vi "Handle Error.vi"(8 "error in (no error)":errorcluster, 11 "Abstract Display Console in":refnum<class "Abstract Display Console.lvclass">) -> (0 "error out":errorcluster, 2 "stop actor?":bool=TRUE, 3 "Abstract Display Console out":refnum<class "Abstract Display Console.lvclass">)   [LabVIEW 2019, in "Abstract Display Console Actor.lvlib" / "Abstract Display Console.lvclass"]
doc: "(<B>Filename</B>: Actor Framework.lvlib:Actor.lvclass:Handle Error.vi)\n\nDefines how the actor handles an error that occurred while processing a message. By default, this method does nothing except stop the actor."
uses:
  Abstract Display Console.lvclass
  C:/Program Files (x86)/National Instruments/LabVIEW 2019/vi.lib/ActorFramework/Actor/Actor.lvclass
  <vilib>/ActorFramework/Actor/Actor.lvclass/Actor.ctl
  Elevator Controller Actor/Elevator Controller Messages/Centrize Error Handler Msg/Centrize Error Handler Msg.lvclass/Centrize Error Handler Msg.ctl
  <vilib>/ActorFramework/Message Enqueuer/Message Enqueuer.lvclass/Message Enqueuer.ctl
  <vilib>/ActorFramework/Message Enqueuer/Enqueue.vi
  Elevator Controller Actor/Elevator Controller Messages/Centrize Error Handler Msg/Centrize Error Handler Msg.lvclass
  C:/Program Files (x86)/National Instruments/LabVIEW 2019/vi.lib/ActorFramework/Message/Message.lvclass
  <vilib>/ActorFramework/Message Priority Queue/Priority Enqueue.vi
  <vilib>/ActorFramework/Actor/Actor.lvclass
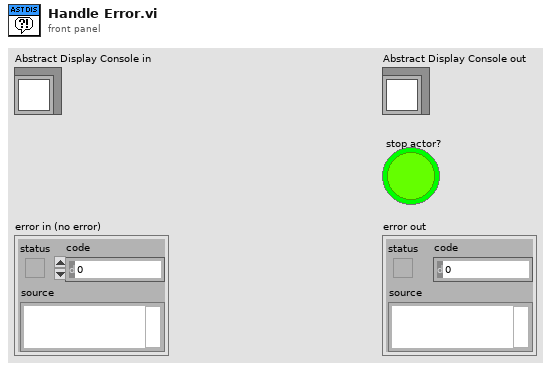
[diagram p1: front panel]
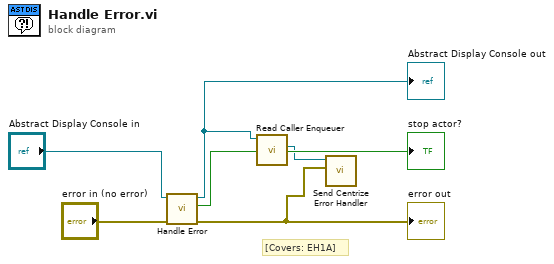
[diagram p0: block diagram]
diagram:
  # "[Covers: EH1A]"
  n1 = call-parent "Handle Error.vi"("error in (no error)"="error in (no error)", "Actor in"="Abstract Display Console in") -> ("error out"=w1:errorcluster, "stop actor?"=→"stop actor?":bool, "Actor out"=w2:refnum<class "Abstract Display Console.lvclass">)  [unwired: 7 in]
  "Abstract Display Console out" <- w2
  "error out" <- w1
  n2 = call <vilib>:"Read Caller Enqueuer.vi"("Actor"=w2) -> ("Caller Enqueuer"=w3:refnum<class "Message Enqueuer.lvclass">)  [unwired: 10 in]
  n3 = call "Send Centrize Error Handler.vi"("Error"=w1, "Message Enqueuer"=w3) -> ()  [unwired: 8 in, 2 out]
